vi "VI_UsingSharedVariable.vi"() -> (3 "SharedVariable":dbl)   [LabVIEW 2012]
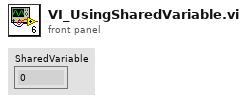
[diagram p1: front panel]
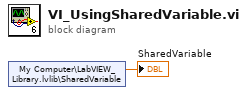
[diagram p0: block diagram]
diagram:
  n1 = shared-variable "My Computer\\LabVIEW_Library.lvlib\\SharedVariable"() -> (→"SharedVariable":dbl)  [unwired: 1 in, 1 out]
